vi "Register for Events (Object Array).vi"(8 "error in (no error)":errorcluster, 9 "PyObject []":refnum<class "PyObject.lvclass">[](array[class]), 11 "JKI_Python_Server in":refnum<class "Server.lvclass">) -> (0 "error out":errorcluster, 1 "Python Event":T1, 3 "JKI_Python_Server out":refnum<class "Server.lvclass">)   [LabVIEW 2020, in "jki_python_bridge.lvlib" / "Server.lvclass"]
uses:
  Server.lvclass
  Type Definitions/Python Method Call - Event Registration.ctl
  Call/Call.lvclass
  Type Definitions/Public Events - Cluster.ctl
  PyObject/PyObject.lvclass
  PyObject/PyObject.lvclass/PyObject.ctl
  Server.lvclass/Server.ctl
  Type Definitions/Python Node.ctl
  <userlib>/_OpenG.lib/error/error.llb/openg_error.lvlib
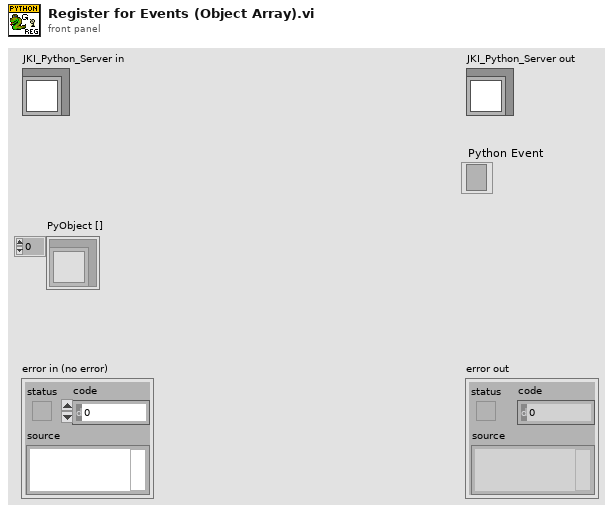
[diagram p1: front panel]
types:
  T1 = typedef "jki_python_bridge.lvlib/Server.lvclass/Python Method Call - Event Registration.ctl" = refnum<event-registration>
  T2 = typedef "jki_python_bridge.lvlib/Server.lvclass/Python Node.ctl" = cluster{"Name":string, "Python Method Call":refnum<user-event>, "Call Handle":refnum<class "PyObject.lvclass">}
  T3 = typedef "jki_python_bridge.lvlib/Server.lvclass/Public Events - Cluster.ctl" = cluster{"Stop Nodes":refnum<user-event>}
  T4 = typedef "jki_python_bridge.lvlib/Server.lvclass/Class Private Data - Cluster.ctl" = cluster{"TCP Server Refnum":refnum<class "JKI TCP Server.lvclass">, "TCP port (50007)":u16, "max connections (0: no limit)":u32, "net address (0: Listen on All Adaptors)":u32, "Nodes":T2[], "Public Events":T3}
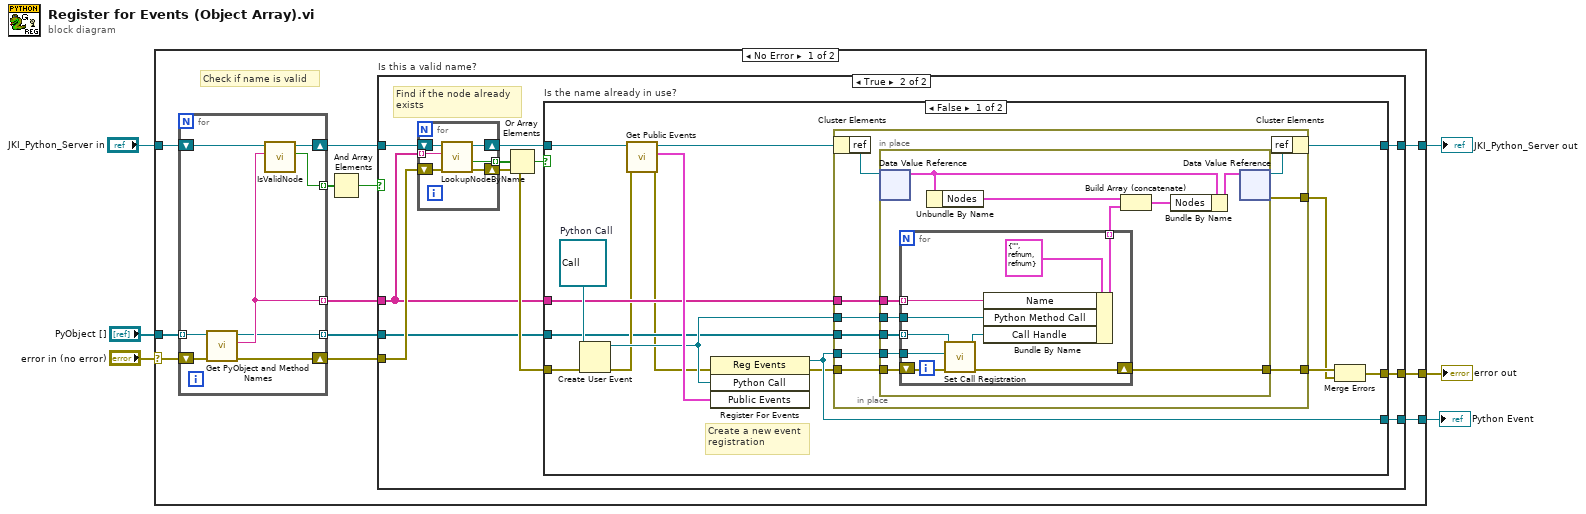
[diagram p0: block diagram]
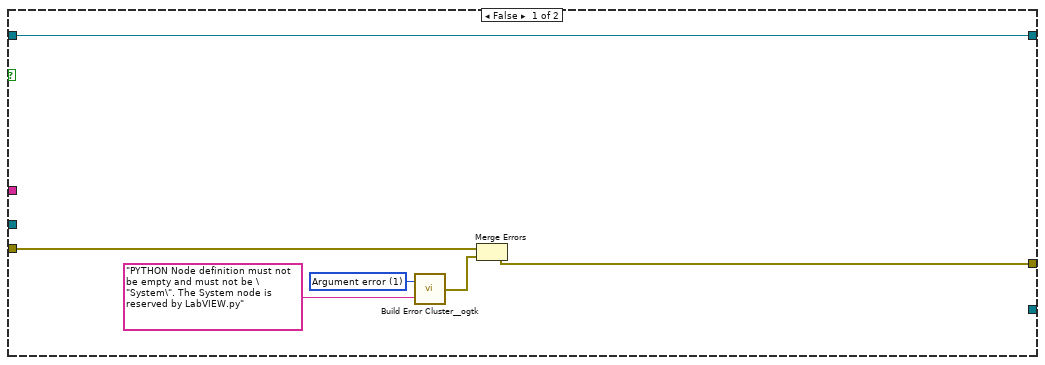
[diagram p2: hidden frame]
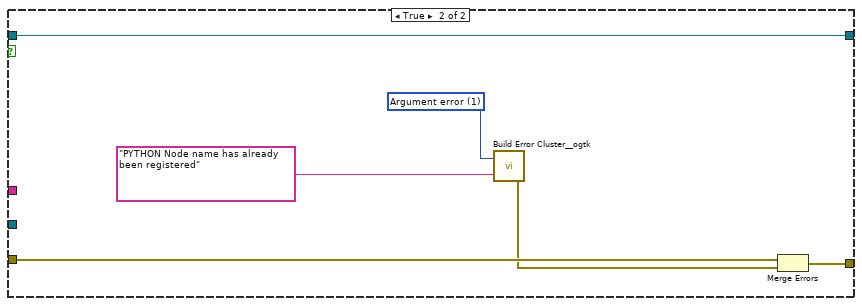
[diagram p3: hidden frame]
diagram:
  n1 = case shown="No Error" "error in (no error)" {
    selector: "error in (no error)" -> [w9 w102]
    tunnel: [w14 w102] -> w5
    tunnel: [w15 w101] -> w3
    tunnel: "JKI_Python_Server in" -> [w18 w101]
    tunnel: [w13 _] -> w2
    tunnel: "PyObject []" -> [w12 _]
    frame No Error {
      # "Check if name is valid"
      n2 = for {
        tunnel: [w24] -> w16 mode=indexing
        tunnel: w12 -> [w23] mode=indexing
        tunnel: [w22] -> w11 mode=indexing
        tunnel: [w21] -> w10 mode=indexing
        shift-right: [w19] -> w8
        shift-left: w9 -> [w20]
        shift-right: [w25] -> w17
        shift-left: w18 -> [w26]
        n3 = call "Get PyObject and Method Names.vi"("error in (no error)"=w20, "Node in"=w23) -> ("error out"=w19:errorcluster, "Object Name"=w22:string, "Node out"=w21:refnum<class "PyObject.lvclass">)  [unwired: 6 in, 1 out]
        n4 = call "IsValidNode.vi"("Node Name"=w22, "Server in"=w26) -> ("Valid Node Definition?"=w24:bool, "Server out"=w25:refnum<class "Server.lvclass">)  [unwired: 8 in]
      }
      n5 = And Array Elements(Boolean array=w16) -> (logical AND=w7:bool)
      n6 = case "Is this a valid name?" shown="True" w7 {
        tunnel: w17 -> [w30 w42]
        tunnel: [w30 w43] -> w15
        tunnel: w11 -> [_ w34]
        tunnel: [_ w39] -> w13
        tunnel: w8 -> [w29 w38]
        tunnel: [w27 w36] -> w14
        tunnel: w10 -> [_ w35]
        frame False {
          w31 = 1 items=["No error", "Argument error", "Memory is full", "Out of zone", "End of file", "File already open", "Generic file I/O error", "File not found", "File permission error", "Disk is full", "Duplicate path", "Too many files open", "System feature not enabled", "Resource file not found", "Cannot add resource", "Resource not found", "Image not found", "Image memory error", "Pen does not exist", "Config type invalid", "Config token not found", "Config parse error", "Config memory error", "Bad external code format", "Bad external code offset", "External code not present", "Null window", "Destroy window error", "Null menu", "Print aborted", "Bad print record", "Print driver error", "Windows error during printing", "Memory error during printing", "Print dialog error", "Generic print error", "Invalid device refnum", "Device not found", "Device parameter error", "Device unit error", "Cannot open device", "Device call aborted", "Generic error", "Cancelled by user", "Object ID too low", "Object ID too high", "Object not in heap", "Unknown heap", "Unknown object (invalid DefProc)", "Unknown object (DefProc not in table)", "Message out of range", "Invalid (null) method", "Unknown message", "Manager call not supported", "Bad address", "Network operation in progress", "Network operation timed out", "Connection is busy", "Network attribute not supported", "Network error", "Address in use", "System out of memory", "Connection aborted", "Connection refused", "Not connected", "Already connected", "Connection closed", "Initialization error (interapplication manager)", "Bad occurrence", "Wait on unbound occurrence handler", "Occurrence queue overflow", "Datalog type conflict", "Unused", "Unrecognized type (interapplication manager)", "Memory corrupt", "Failed to make temporary DLL", "Old CIN version", "Drag socket not found", "Failed to load drop-object", "Failed to register OLE object", "Failed to release OLE object", "Format specifier type mismatch", "Unknown format specifier", "Too few format specifiers", "Too many format specifiers", "Scan failed", "Newer CIN version", "Error converting to variant", "Runtime menu error", "Password tampered", "Variant attribute not found", "Incompatible variant data type", "Event data is not available", "Event Store is not present", "Occurrence is not found", "Event Queue is not created", "Event info is not available", "Refnum passed is NULL", "Error retrieving Class GUID", "Error retrieving CoClass GUID", "Error retrieving TypeLib GUID.", "Bad built application magic bytes.", "Specific driver is different from the specific driver associated with the Logical Name.", "There is no session opened to the class driver.", "Max Error", "MAX - Error with config objects", "MAX - Error loading configuration", "MAX - Group not supported"]
          n7 = call <userlib>:"Build Error Cluster__ogtk.vi"("String to Prepend to source (\"\")"="PYTHON Node definition must not be empty and must not be \"System\". The System node is reserved by LabVIEW.py", "code"=w31) -> ("error out"=w28:errorcluster)
          n8 = Merge Errors(w29, w28) -> (w27:errorcluster)
        }
        frame True {
          # "Find if the node already\nexists"
          n9 = for {
            tunnel: [w47] -> w40 mode=indexing
            tunnel: w34 -> [w44] mode=indexing
            shift-right: [w45] -> w37
            shift-left: w38 -> [w46]
            shift-right: [w48] -> w41
            shift-left: w42 -> [w49]
            n10 = call "LookupNodeByName.vi"("error in (no error)"=w46, "Python Node Name"=w44, "Server in"=w49) -> ("error out"=w45:errorcluster, "Found?"=w47:bool, "Server out"=w48:refnum<class "Server.lvclass">)  [unwired: 5 in, 1 out]
          }
          n11 = Or Array Elements(Boolean array=w40) -> (logical OR=w33:bool)
          n12 = case "Is the name already in use?" shown="False" w33 {
            tunnel: [w61 w98] -> w43
            tunnel: w41 -> [w63 w98]
            tunnel: w34 -> [w60 _]
            tunnel: [w53 _] -> w39
            tunnel: w37 -> [w57 w97]
            tunnel: [w58 w96] -> w36
            tunnel: w35 -> [w55 _]
            frame False {
              w64 = refnum<class "Call.lvclass"> refnum  # Python Call
              # "Create a new event\nregistration"
              n13 = Create User Event(user event datatype=w64, error in=w57) -> (user event=w59:refnum<user-event>, error out=w56:errorcluster)
              n14 = call "Get Public Events.vi"("error in (no error)"=w56, "JKI_Python_Server in"=w63) -> ("error out"=w51:errorcluster, "Public Events"=w65:T3, "JKI_Python_Server out"=w62:refnum<class "Server.lvclass">)  [unwired: 7 in]
              n15 = register-events(error in=w51, w59, w65) -> (reference out=w53:refnum<event-registration>, error out=w50:errorcluster)  [unwired: 1 in]
              n16 = in-place {
                in-place-border: w60 -> [w72]
                in-place-border: [w71] -> w52
                in-place-border: w59 -> [w70]
                in-place-border: w55 -> [w69]
                in-place-border: w50 -> [w68]
                in-place-border: [w67] -> w54
                in-place-border: w53 -> [w66]
                n17 = in-place-cluster #1(w62) -> ("ref"=w74:refnum<data-value>)
                n18 = in-place {
                  in-place-border: w72 -> [w81]
                  in-place-border: w70 -> [w80]
                  in-place-border: w69 -> [w78]
                  in-place-border: w68 -> [w77]
                  in-place-border: [w76] -> w67
                  in-place-border: w66 -> [w75]
                  n19 = in-place-dvr #2(w74) -> (w84:T4)  [unwired: 1 out]
                  n20 = for {
                    tunnel: w81 -> [w93] mode=indexing
                    tunnel: w80 -> [w92]
                    tunnel: [w91] -> w79 mode=indexing
                    tunnel: w78 -> [w90] mode=indexing
                    tunnel: w75 -> [w87]
                    shift-right: [w88] -> w76
                    shift-left: w77 -> [w89]
                    n21 = call "Set Call Registration.vi"("error in (no error)"=w89, "Call Registration"=w87, "Node in"=w90) -> ("error out"=w88:errorcluster, "Node out"=w86:refnum<class "PyObject.lvclass">)  [unwired: 7 in]
                    n22 = Bundle By Name(cluster=T2 {"Name"="", "Python Method Call"=refnum, "Call Handle"=refnum} ("PYTHON Node"), "Name"=w93, "Python Method Call"=w92, "Call Handle"=w86) -> (w91:T2)
                  }
                  n23 = Unbundle By Name(w84) -> ("Nodes"=w83:T2[])
                  n24 = Build Array (concatenate)(w83, w79) -> (w82:T2[])
                  n25 = Bundle By Name(cluster=w84, "Nodes"=w82) -> (w85:T4)
                  n26 = in-place-dvr #2(w85) -> (w73:refnum<data-value>, w71:errorcluster)
                }
                n27 = in-place-cluster #1("ref"=w73) -> (w61:refnum<class "Server.lvclass">)
              }
              n28 = Merge Errors(w54, w52) -> (w58:errorcluster)
            }
            frame True {
              w99 = 1 items=["No error", "Argument error", "Memory is full", "Out of zone", "End of file", "File already open", "Generic file I/O error", "File not found", "File permission error", "Disk is full", "Duplicate path", "Too many files open", "System feature not enabled", "Resource file not found", "Cannot add resource", "Resource not found", "Image not found", "Image memory error", "Pen does not exist", "Config type invalid", "Config token not found", "Config parse error", "Config memory error", "Bad external code format", "Bad external code offset", "External code not present", "Null window", "Destroy window error", "Null menu", "Print aborted", "Bad print record", "Print driver error", "Windows error during printing", "Memory error during printing", "Print dialog error", "Generic print error", "Invalid device refnum", "Device not found", "Device parameter error", "Device unit error", "Cannot open device", "Device call aborted", "Generic error", "Cancelled by user", "Object ID too low", "Object ID too high", "Object not in heap", "Unknown heap", "Unknown object (invalid DefProc)", "Unknown object (DefProc not in table)", "Message out of range", "Invalid (null) method", "Unknown message", "Manager call not supported", "Bad address", "Network operation in progress", "Network operation timed out", "Connection is busy", "Network attribute not supported", "Network error", "Address in use", "System out of memory", "Connection aborted", "Connection refused", "Not connected", "Already connected", "Connection closed", "Initialization error (interapplication manager)", "Bad occurrence", "Wait on unbound occurrence handler", "Occurrence queue overflow", "Datalog type conflict", "Unused", "Unrecognized type (interapplication manager)", "Memory corrupt", "Failed to make temporary DLL", "Old CIN version", "Drag socket not found", "Failed to load drop-object", "Failed to register OLE object", "Failed to release OLE object", "Format specifier type mismatch", "Unknown format specifier", "Too few format specifiers", "Too many format specifiers", "Scan failed", "Newer CIN version", "Error converting to variant", "Runtime menu error", "Password tampered", "Variant attribute not found", "Incompatible variant data type", "Event data is not available", "Event Store is not present", "Occurrence is not found", "Event Queue is not created", "Event info is not available", "Refnum passed is NULL", "Error retrieving Class GUID", "Error retrieving CoClass GUID", "Error retrieving TypeLib GUID.", "Bad built application magic bytes.", "Specific driver is different from the specific driver associated with the Logical Name.", "There is no session opened to the class driver.", "Max Error", "MAX - Error with config objects", "MAX - Error loading configuration", "MAX - Group not supported"]
              n29 = call <userlib>:"Build Error Cluster__ogtk.vi"("String to Prepend to source (\"\")"="PYTHON Node name has already been registered", "code"=w99) -> ("error out"=w95:errorcluster)
              n30 = Merge Errors(w97, w95) -> (w96:errorcluster)
            }
          }
        }
      }
    }
    frame Error {
    }
  }
  "error out" <- w5
  "JKI_Python_Server out" <- w3
  "Python Event" <- w2
